vi "Main GUI.vi"() -> ()   [LabVIEW 2018]
uses:
  Button Class/Button Handler State.ctl
  Button Class/TCP Message Payload.ctl
  Button Class/Button.lvclass
panel:
  out "T3H10":bool
  out "T3H8/H9":bool
  out "T3H6/H7":bool
  out "T2F8/F9":bool
  out "T1A1/A2":bool
  out "T1A13/A14":bool
  out "T1A11/A12":bool
  out "T1A9/A10":bool
  out "T1A8":bool
  out "T1A7":bool
  out "T1A5/A6":bool
  out "T1A3/A4":bool
  out "T1F3":bool
  out "T1F1/F2":bool
  out "T1E11/E12":bool
  out "T1E9/E10":bool
  out "T1E7/E8":bool
  out "T1E5/E6":bool
  out "T1E3/E4":bool
  out "T1E1/E2":bool
  out "T1D13/D14":bool
  out "T1D11/D12":bool
  out "T1D9/D10":bool
  out "T1D8":bool
  out "T1D7":bool
  out "T1D5/D6":bool
  out "T1D3/D4":bool
  out "T1D1/D2":bool
  out "T1C11/C12":bool
  out "T1C9/C10":bool
  out "T1C7/C8":bool
  out "T1C5/C6":bool
  out "T1C3/C4":bool
  out "T1C1/C2":bool
  out "T1B13/B14":bool
  out "T1B11/B12":bool
  out "T1B9/B10":bool
  out "T1B8":bool
  out "T1B7":bool
  out "T1B5/B6":bool
  out "T1B3/B4":bool
  out "T1B1/B2":bool
  out "T2A1/A2":bool
  out "T2A13/A13":bool
  out "T2A11/A12":bool
  out "T2A9/A10":bool
  out "T2A8":bool
  out "T2A7":bool
  out "T2A5/A6":bool
  out "T2A3/A4":bool
  out "T2G3/G4":bool
  out "T2G1/G2":bool
  out "T2F6/F7":bool
  out "T2F4/F5":bool
  out "T2F3":bool
  out "T2F1/F2":bool
  out "T2E13/E14":bool
  out "T2E11/E12":bool
  out "T2E9/E10":bool
  out "T2E8":bool
  out "T2E7":bool
  out "T2E5/E6":bool
  out "T2E3/E4":bool
  out "T2D13/D14":bool
  out "T2D11/D12":bool
  out "T2D9/D10":bool
  out "T2D8":bool
  out "T2D7":bool
  out "T2D5/D6":bool
  out "T2D3/D4":bool
  out "T2D1/D2":bool
  out "T2C13/C14":bool
  out "T2C11/C12":bool
  out "T2C9/C10":bool
  out "T2C8":bool
  out "T2C7":bool
  out "T2C5/C6":bool
  out "T2C3/C4":bool
  out "T2C1/C2":bool
  out "T2B13/B14":bool
  out "T2B11/B12":bool
  out "T2B9/B10":bool
  out "T2B8":bool
  out "T2B7":bool
  out "T2B5/B6":bool
  out "T2B3/B4":bool
  out "T2B1/B2":bool
  in  "Quit":bool
  out "T3A1/A2":bool
  out "T3A13/A14":bool
  out "T3A11/A12":bool
  out "T3A9/A10":bool
  out "T3A8":bool
  out "T3A7":bool
  out "T3A5/A6":bool
  out "T3A3/A4":bool
  out "I3":bool
  out "I2":bool
  out "I1":bool
  out "T3H5":bool
  out "T3H3/H4":bool
  out "T3H1/H2":bool
  out "T3G13/G14":bool
  out "T3G11/G12":bool
  out "T3G9/G10":bool
  out "T3G8":bool
  out "T3G7":bool
  out "T3G5/G6":bool
  out "T3G3/G4":bool
  out "T3G1/G2":bool
  out "T3F13/F14":bool
  out "T3F11/F12":bool
  out "T3F9/F10":bool
  out "T3F8":bool
  out "T3F7":bool
  out "T3F5/F6":bool
  out "T3F3/F4":bool
  out "T3F1/F2":bool
  out "T3E13/E14":bool
  out "T3E11/E12":bool
  out "T3E9/E10":bool
  out "T3E8":bool
  out "T3E7":bool
  out "T3E5/E6":bool
  out "T3E3/E4":bool
  out "T3E1/E2":bool
  out "T3D13/D14":bool
  out "T3D11/D12":bool
  out "T3D9/D10":bool
  out "T3D8":bool
  out "T3D7":bool
  out "T3D5/D6":bool
  out "T3D3/D4":bool
  out "T3D1/D2":bool
  out "T3C13/C14":bool
  out "T3C11/C12":bool
  out "T3C9/C10":bool
  out "T3C8":bool
  out "T3C7":bool
  out "T3C5/C6":bool
  out "T3C3/C4":bool
  out "T3C1/C2":bool
  out "T3B13/B14":bool
  out "T3B11/B12":bool
  out "T3B9/B10":bool
  out "T3B8":bool
  out "T3B7":bool
  out "T3B5/B6":bool
  out "T3B3/B4":bool
  out "T3B1/B2":bool
  out "error out":errorcluster
  in  "error in (no error)":errorcluster
  # "A1/A2"
  # "A3/A4"
  # "A5/A6"
  # "A7"
  # "A8"
  # "A9/A10"
  # "A11/A12"
  # "A13/A14"
  # "A1/A2"
  # "A3/A4"
  # "A5/A6"
  # "A7"
  # "A8"
  # "A9/A10"
  # "A11/A12"
  # "A13/A14"
  # "B1/B2"
  # "B3/B4"
  # "B5/B6"
  # "B5/B6"
  # "B7"
  # "B8"
  # "B9/B10"
  # "B11/B12"
  # "B13/B14"
  # "B1/B2"
  # "B3/B4"
  # "B5/B6"
  # "B5/B6"
  # "B7"
  # "B8"
  # "B9/B10"
  # "B11/B12"
  # "B13/B14"
  # "C1/C2"
  # "C3/C4"
  # "C5/C6"
  # "C7"
  # "C8"
  # "C9/C10"
  # "C11/C12"
  # "C13/C14"
  # "A1/A2"
  # "A3/A4"
  # "A5/A6"
  # "A7"
  # "A8"
  # "A9/A10"
  # "A11/A12"
  # "A13/A14"
  # "C1/C2"
  # "C3/C4"
  # "C5/C6"
  # "C7"
  # "C8"
  # "C9/C10"
  # "C11/C12"
  # "C13/C14"
  # "D1/D2"
  # "D3/D4"
  # "D5/D6"
  # "D7"
  # "D8"
  # "D9/D10"
  # "D11/D12"
  # "D13/D14"
  # "B1/B2"
  # "B3/B4"
  # "B5/B6"
  # "B5/B6"
  # "B7"
  # "B8"
  # "B9/B10"
  # "B11/B12"
  # "B13/B14"
  # "E1/E2"
  # "E3/E4"
  # "E5/E6"
  # "E7"
  # "E8"
  # "E9/E10"
  # "E11/E12"
  # "E13/E14"
  # "D1/D2"
  # "D3/D4"
  # "D5/D6"
  # "D7"
  # "D8"
  # "D9/D10"
  # "D11/D12"
  # "D13/D14"
  # "C1/C2"
  # "C3/C4"
  # "C5/C6"
  # "C7/C8"
  # "C9/C10"
  # "C11/C12"
  # "F1/F2"
  # "F3/F4"
  # "F5/F6"
  # "F7"
  # "F8"
  # "F9/F10"
  # "F11/F12"
  # "F13/F14"
  # "E3/E4"
  # "E5/E6"
  # "E7"
  # "E8"
  # "E9/E10"
  # "E11/E12"
  # "E13/E14"
  # "G1/G2"
  # "G3/G4"
  # "G5/G6"
  # "G7"
  # "G8"
  # "G9/G10"
  # "G11/G12"
  # "G13/G14"
  # "D1/D2"
  # "D3/D4"
  # "D5/D6"
  # "D7"
  # "D8"
  # "D9/D10"
  # "D11/D12"
  # "D13/D14"
  # "F1/F2"
  # "F3"
  # "F4/F5"
  # "F6/F7"
  # "F8/F9"
  # "E1/E2"
  # "E7/E8"
  # "E9/E10"
  # "E11/E12"
  # "E3/E4"
  # "E5/E6"
  # "H1/H2"
  # "H3/H4"
  # "H5"
  # "H6/H7"
  # "H8/H9"
  # "H10"
  # "G1/G2"
  # "G3/G4"
  # "I1/I2"
  # "I3/I4"
  # "I5"
  # "F1/F2"
  # "F3/F4"
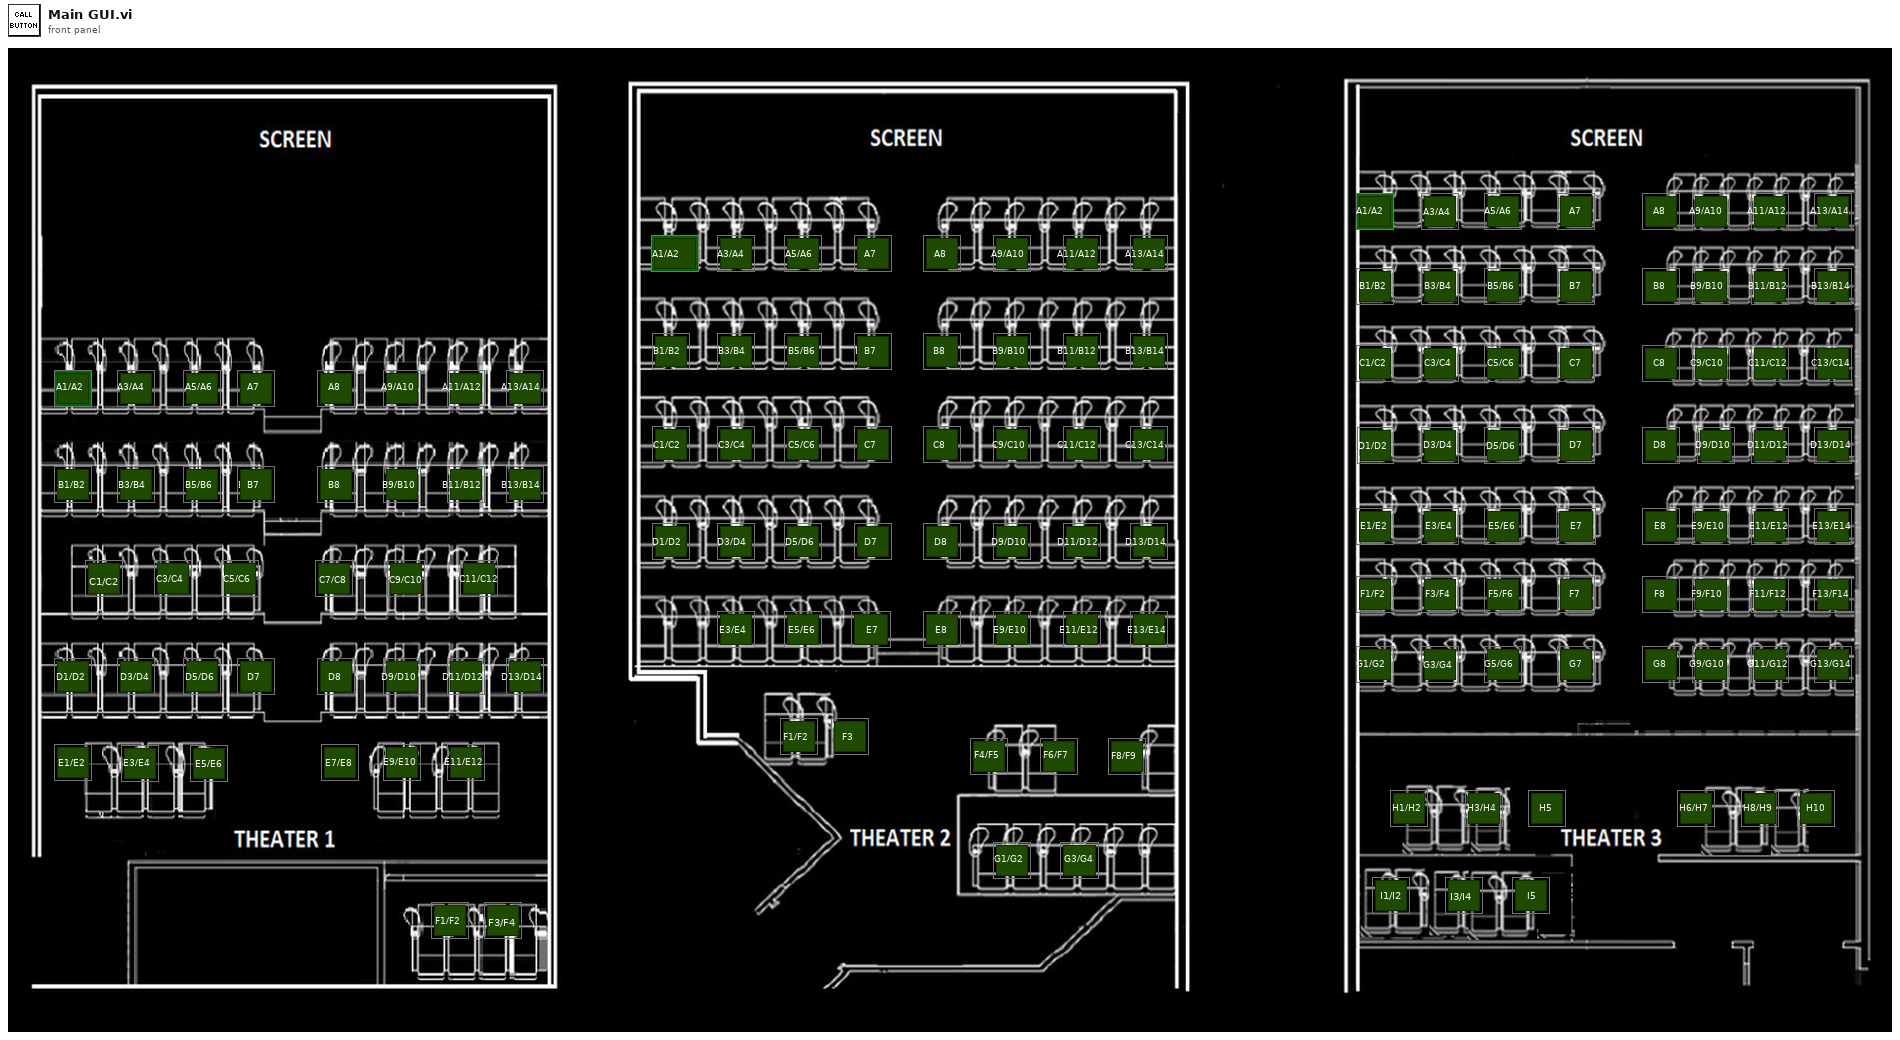
[diagram p1: front panel]
types:
  T1 = typedef "TCP Message Payload.ctl" = cluster{"ID":string, "First Active":timestamp, "Button State":bool}
  T2 = typedef "Button Handler State.ctl" = enum16{"Initialize", "Check Active", "Update Colors", "Message Check"}
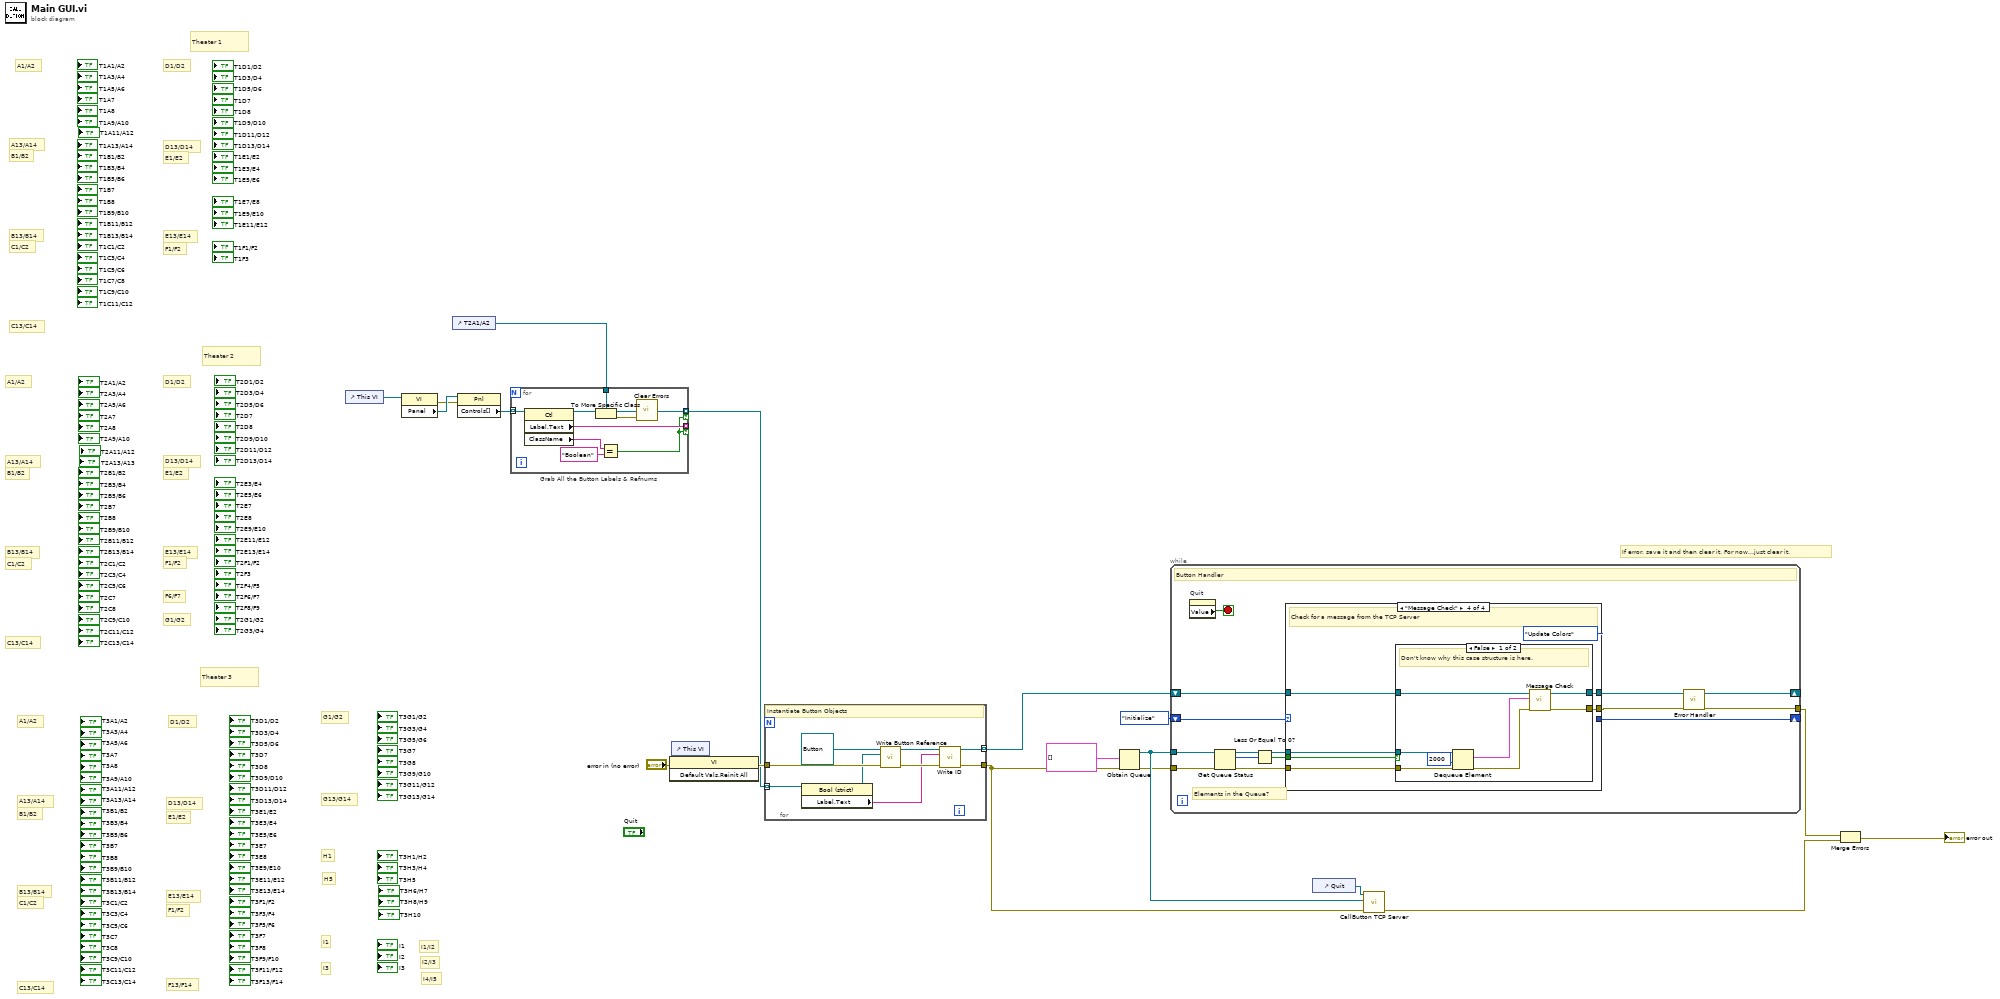
[diagram p0: block diagram]
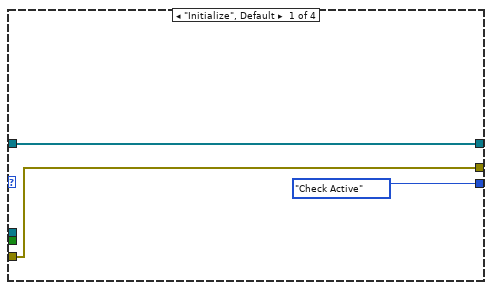
[diagram p2: hidden frame]
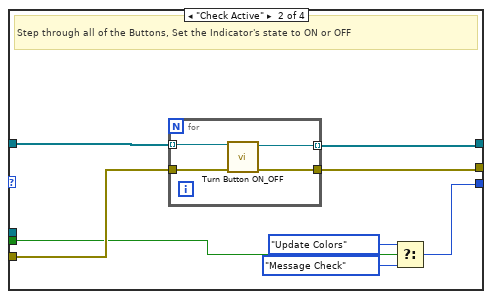
[diagram p3: hidden frame]
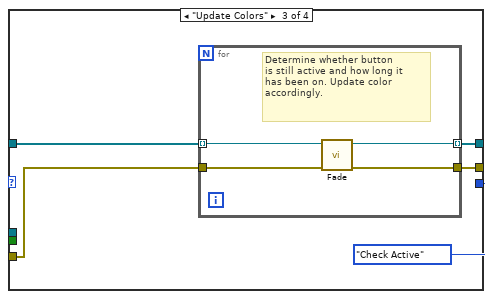
[diagram p4: hidden frame]
diagram:
  # "If error, save it and then clear it. For now...just clear it."
  # "I4/I5"
  # "I2/I3"
  # "I1/I2"
  # "C13/C14"
  # "C1/C2"
  # "B13/B14"
  # "B1/B2"
  # "A13/A14"
  # "F1/F2"
  # "E13/E14"
  # "E1/E2"
  # "D1/D2"
  # "D13/D14"
  # "A1/A2"
  # "Theater 1"
  # "G1/G2"
  # "F6/F7"
  # "F1/F2"
  # "E13/E14"
  # "C13/C14"
  # "C1/C2"
  # "B13/B14"
  # "E1/E2"
  # "D1/D2"
  # "D13/D14"
  # "B1/B2"
  # "A13/A14"
  # "A1/A2"
  # "Theater 2"
  # "G13/G14"
  # "H5"
  # "I3"
  # "I1"
  # "H1"
  # "G1/G2"
  # "F13/F14"
  # "F1/F2"
  # "E13/E14"
  # "E1/E2"
  # "D1/D2"
  # "D13/D14"
  # "C13/C14"
  # "C1/C2"
  # "B13/B14"
  # "B1/B2"
  # "A13/A14"
  # "A1/A2"
  # "Theater 3"
  n1 = control-ref of="This VI"() -> (w6:refnum<vi>)
  n2 = property class="VI"(reference=w6) -> (error out=w4:errorcluster, "Panel"=w5:refnum<vi>)  [unwired: 1 in, 1 out]
  n3 = control-ref of="T2A1/A2"() -> (w2:refnum<vi>)
  n4 = property class="Pnl"(reference=w5, error in=w4) -> ("Controls[]"=w3:refnum<vi>[])  [unwired: 2 out]
  n5 = for "Grab All the Button Labels & Refnums" {
    tunnel: w3 -> [w28] mode=indexing
    tunnel: [w21] -> w1 mode=indexing if=w24
    tunnel: [w25] -> _ mode=indexing if=w24
    tunnel: w2 -> [w22]
    n6 = property class="Ctl"(reference=w28) -> (reference out=w23:refnum<vi>, "Label.Text"=w25:string, "ClassName"=w26:string)  [unwired: 1 in, 1 out]
    n7 = To More Specific Class(target class=w22, reference=w23) -> (specific class reference=w21:refnum<vi>, error out=w20:errorcluster)  [unwired: 1 in]
    n8 = Equal?(x=w26, y="Boolean" ("regular expression")) -> (x = y?=w24:bool)
    n9 = call <vilib>:"Clear Errors.vi"("error in (no error)"=w20) -> ()  [unwired: 5 in, 2 out]
  }
  n10 = control-ref of="This VI"() -> (w19:refnum<vi>)
  n11 = invoke class="VI" method="Default Vals.Reinit All"(reference=w19, error in="error in (no error)") -> (error out=w17:errorcluster)  [unwired: 1 in, 2 out]
  n12 = for {
    tunnel: w1 -> [w31] mode=indexing
    tunnel: [w33] -> w12 mode=indexing
    tunnel: w17 -> [w36]
    tunnel: [w32] -> w8
    # "Instantiate Button Objects"
    n13 = property class="Bool (strict)"(reference=w31) -> (reference out=w30:refnum<vi>, "Label.Text"=w29:string)  [unwired: 1 in, 1 out]
    n14 = call-dynamic "Write Button Reference.vi"("error in (no error)"=w36, "Button Reference"=w30, "Button in"=refnum<class "Button.lvclass"> refnum ("Button.lvclass")) -> ("error out"=w34:errorcluster, "Button out"=w35:refnum<class "Button.lvclass">)  [unwired: 7 in]
    n15 = call-dynamic "Write ID.vi"("error in (no error)"=w34, "ID"=w29, "Button in"=w35) -> ("error out"=w32:errorcluster, "Button out"=w33:refnum<class "Button.lvclass">)  [unwired: 7 in]
  }
  n16 = Obtain Queue(element data type=T1[] [] ("element"), error in (no error)=w8) -> (queue out=w11:refnum<queue>, error out=w7:errorcluster)  [unwired: 3 in, 1 out]
  n17 = while {
    shift-right: [w49] -> _
    shift-left: Button_Handler_State."Initialize" -> [w50]
    tunnel: [w38] -> w15
    shift-right: [w46] -> _
    shift-left: w12 -> [w47]
    tunnel: w11 -> [w45]
    tunnel: w7 -> [w42]
    stop <- w48 stop-if-true
    # "Elements in the Queue?"
    # "Button Handler"
    n18 = property on="Quit" class="Bool (strict)"() -> ("Value"=w48:bool)  [unwired: 2 in, 2 out]
    n19 = Get Queue Status(queue=w45, error in (no error)=w42) -> (queue out=w44:refnum<queue>, error out=w41:errorcluster, # elements in queue=w40:i32)  [unwired: 1 in, 5 out]
    n20 = Less Or Equal To 0?(x=w40) -> (x <= 0?=w43:bool)
    n21 = case shown="\"Message Check\"" w50 {
      tunnel: w47 -> [w52 w61 w70 w81]
      tunnel: [Button_Handler_State."Check Active" w57 Button_Handler_State."Check Active" Button_Handler_State."Update Colors"] -> w49
      tunnel: [w51 w60 w69 w80] -> w39
      tunnel: [w52 w56 w67 w78] -> w46
      tunnel: w44 -> [_ _ _ w77]
      tunnel: w43 -> [_ w54 _ w76]
      tunnel: w41 -> [w51 w55 w66 w75]
      frame "Initialize", Default {
      }
      frame "Check Active" {
        # "Step through all of the Buttons, Set the Indicator's state to ON or OFF"
        n22 = for {
          tunnel: w61 -> [w65] mode=indexing
          tunnel: [w64] -> w60
          tunnel: [w63] -> w56 mode=indexing
          tunnel: w55 -> [w62]
          n23 = call "Turn Button ON_OFF.vi"("error in (no error)"=w62, "Button in"=w65) -> ("error out"=w64:errorcluster, "Button out"=w63:refnum<class "Button.lvclass">)  [unwired: 8 in]
        }
        n24 = Select(t=Button_Handler_State."Update Colors", s=w54, f=Button_Handler_State."Message Check") -> (s? t:f=w57:T2)
      }
      frame "Update Colors" {
        n25 = for {
          tunnel: w70 -> [w73] mode=indexing
          tunnel: [w74] -> w69
          tunnel: [w72] -> w67 mode=indexing
          tunnel: w66 -> [w71]
          # "Determine whether button\nis still active and how long it\nhas been on. Update color \naccordingly."
          n26 = call "Fade.vi"("error in (no error)"=w71, "Button in"=w73) -> ("error out"=w74:errorcluster, "Button out"=w72:refnum<class "Button.lvclass">)  [unwired: 8 in]
        }
      }
      frame "Message Check" {
        # "Check for a message from the TCP Server"
        n27 = case shown="False" w76 {
          tunnel: w81 -> [w89 w91]
          tunnel: [w88 w90] -> w80
          tunnel: [w87 w91] -> w78
          tunnel: w77 -> [w86 _]
          tunnel: w75 -> [w83 w90]
          frame False {
            # "Don't know why this case structure is here."
            n28 = Dequeue Element(queue=w86, timeout in ms (-1)=2000, error in (no error)=w83) -> (element=w84:T1[], error out=w82:errorcluster)  [unwired: 2 out]
            n29 = call "Message Check.vi"("error in (no error)"=w82, "ID & Time"=w84, "Button Object Array In"=w89) -> ("error out"=w88:errorcluster, "Button Object Array Out"=w87:refnum<class "Button.lvclass">[])  [unwired: 7 in]
          }
          frame True {
          }
        }
      }
    }
    n30 = call "Error Handler.vi"("error in (no error)"=w39) -> ("error out (no error)"=w38:errorcluster)  [unwired: 10 in]
  }
  n31 = control-ref of="Quit"() -> (w9:refnum<vi>)
  n32 = call "CallButton TCP Server.vi"("error in (no error)"=w8, "queue in"=w11, "Boolean in"=w9) -> ("error out"=w13:errorcluster)  [unwired: 8 in]
  n33 = Merge Errors(w15, w13) -> (→"error out":errorcluster)
